vi "CSC_GetCableJacobian_Fast.vi"(8 "error in (no error)":errorcluster, 11 "C-Alex in":refnum<class "CableSerialChain.lvclass">) -> (0 "error out":errorcluster, 2 "Jacobian for Cables":T1, 3 "C-Alex out":refnum<class "CableSerialChain.lvclass">)   [LabVIEW 2015, in "CableSerialChain.lvclass"]
uses:
  CableSerialChain.lvclass
  <vilib>/Analysis/Matrix/Datatypes/RealMatrix.ctl
  CableSerialChain.lvclass/CableSerialChain.ctl
  Body/Force.ctl
  Body/PointOnBody.ctl
  <vilib>/Analysis/BLAS.llb/dnrm2 - Vector 2-Norm (DBL).vi
  <vilib>/Analysis/Matrix/Numeric/Conversions/Array To Matrix - RA2.vi
  Body/Bodies.lvclass
  <vilib>/Analysis/NI_AALBLAS.lvlib
  <vilib>/Analysis/Matrix/NI_Matrix.lvlib
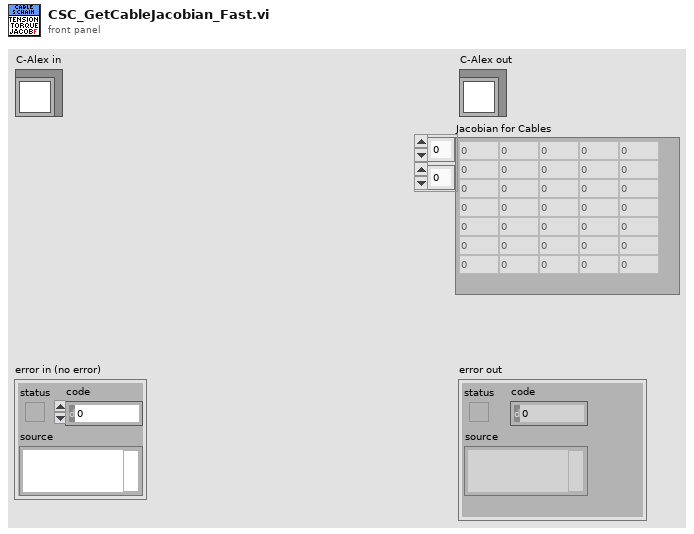
[diagram p1: front panel]
types:
  T1 = typedef "NI_Matrix.lvlib/RealMatrix.ctl" = dbl[][]
  T2 = typedef "Bodies.lvclass/Force.ctl" = cluster{"LocationInLCS":T3, "ForceVector":dbl[]}
  T3 = typedef "Bodies.lvclass/PointOnBody.ctl" = cluster{"Coord4":dbl[], "ID":i32}
  T4 = typedef "CableSerialChain.lvclass/Cable.ctl" = cluster{"RoutingPtsInLCS":T3[], "Cable ID":i32, "ActiveSegments":i32[][]}
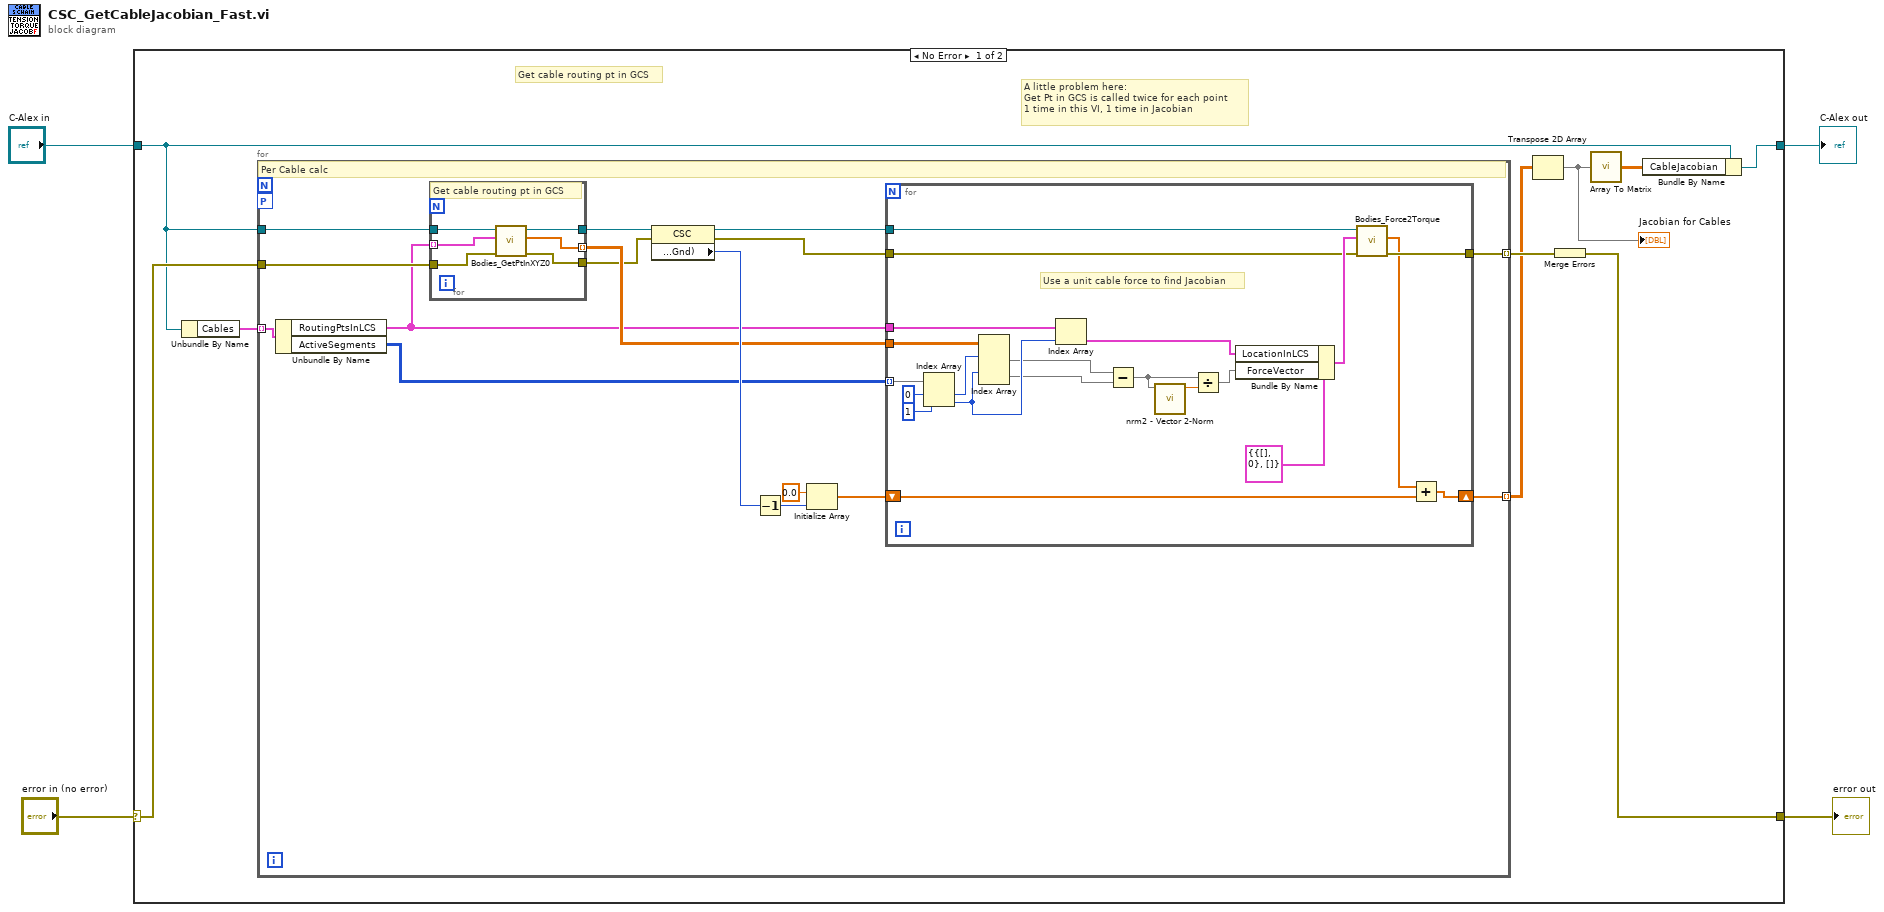
[diagram p0: block diagram]
diagram:
  n1 = case shown="No Error" "error in (no error)" {
    selector: "error in (no error)" -> [w12 w57]
    tunnel: [w8 w57] -> w3
    tunnel: [w7 w58] -> w1
    tunnel: "C-Alex in" -> [w5 w58]
    frame No Error {
      # "Get cable routing pt in GCS"
      # "A little problem here:\nGet Pt in GCS is called twice for each point\n1 time in this VI, 1 time in Jacobian"
      n2 = Unbundle By Name(w5) -> ("Cables"=w13:T4[])
      n3 = for {
        tunnel: w13 -> [w29] mode=indexing
        tunnel: [w17] -> w10 mode=indexing
        tunnel: w12 -> [w24]
        tunnel: [w16] -> w11 mode=indexing
        tunnel: w5 -> [w28]
        workers-P: _ -> [_]
        # "Per Cable calc"
        n4 = Unbundle By Name(w29) -> ("RoutingPtsInLCS"=w22:T3[], "ActiveSegments"=w14:i32[][])
        n5 = for {
          tunnel: w22 -> [w54] mode=indexing
          tunnel: w24 -> [w53]
          tunnel: [w52] -> w20
          tunnel: [w51] -> w23 mode=indexing
          tunnel: w28 -> [w56]
          tunnel: [w55] -> w21
          # "Get cable routing pt in GCS"
          n6 = call "Bodies_GetPtInXYZ0.vi"("error in (no error)"=w53, "Point"=w54, "Bodies.lvclass"=w56) -> ("error out"=w52:errorcluster, "PointInGCS"=w51:dbl[], "Bodies.lvclass 2"=w55:refnum<class "CableSerialChain.lvclass">)  [unwired: 5 in, 1 out]
        }
        n7 = property class="CSC"(reference=w21, error in=w20) -> (reference out=w19:refnum<class "CableSerialChain.lvclass">, error out=w15:errorcluster, "#ofBodies(Inc.Gnd)"=w26:i32)
        n8 = Decrement(x=w26) -> (x-1=w25:i32)
        n9 = Initialize Array(0.0 ("element"), w25) -> (w18:dbl[])
        n10 = for {
          tunnel: w14 -> [w50] mode=indexing
          tunnel: w23 -> [w46]
          tunnel: w22 -> [w45]
          tunnel: w15 -> [w35]
          tunnel: w19 -> [w34]
          tunnel: [w33] -> w16
          shift-right: [w32] -> w17
          shift-left: w18 -> [w30]
          # "Use a unit cable force to find Jacobian"
          n11 = Index Array(array=w50, index #1=0 ("index"), index #2=1 ("index")) -> (element #1=w47:i32, element #2=w44:i32)
          n12 = Index Array(array=w46, index (row) #1=w47, index (row) #2=w44) -> (element #1=w42:dbl[], element #2=w41:dbl[])  [unwired: 2 in]
          n13 = Index Array(array=w45, index=w44) -> (element=w39:T3)
          n14 = Subtract(x=w42, y=w41) -> (x-y=w40:dbl[])
          n15 = call-poly <vilib>:"nrm2 - Vector 2-Norm.vi"("x"=w40) -> ("dnrm2"=w43:dbl)  [unwired: 9 in, 1 out]
          n16 = Divide(x=w40, y=w43) -> (x/y=w38:dbl[])
          n17 = Bundle By Name(cluster=T2 {"LocationInLCS"={"Coord4"=[], "ID"=0}, "ForceVector"=[]} ("Force"), "LocationInLCS"=w39, "ForceVector"=w38) -> (w36:T2)
          n18 = call "Bodies_Force2Torque.vi"("error in (no error)"=w35, "Force"=w36, "Bodies.lvclass"=w34) -> ("error out"=w33:errorcluster, "Torque Vector"=w31:dbl[])  [unwired: 5 in, 2 out]
          n19 = Add(x=w31, y=w30) -> (x+y=w32:dbl[])
        }
      }
      n20 = Transpose 2D Array(2D array=w10) -> (transposed array=w9:dbl[][])
      "Jacobian for Cables" <- w9
      n21 = Merge Errors(w11) -> (w8:errorcluster)
      n22 = call-poly <vilib>:"Array To Matrix.vi"("Real 2D Array"=w9) -> ("Real Matrix"=w6:T1)
      n23 = Bundle By Name(cluster=w5, "CableJacobian"=w6) -> (w7:refnum<class "CableSerialChain.lvclass">)
    }
    frame Error {
    }
  }
  "error out" <- w3
  "C-Alex out" <- w1
